vi "get leafnodes for traverse.vi"(8 "error in":errorcluster caption="错误输入（无错误）", 10 "Data in":refnum<data-value>[](array[refnum]), 11 "Class in":refnum<class "PanelLinkNode.lvclass"> caption="DNL_LabVIEW Object in") -> (0 "error out":errorcluster caption="错误输出", 2 "Data out":refnum<data-value>[](array[refnum]), 3 "Class out":refnum<class "PanelLinkNode.lvclass"> caption="DNL_LabVIEW Object out")   [LabVIEW 2013, in "PanelLinkNode.lvclass"]
uses:
  PanelLinkNode.lvclass
  PanelObject/PanelObject.lvclass
  PanelLinkNode.lvclass/PanelLinkNode.ctl
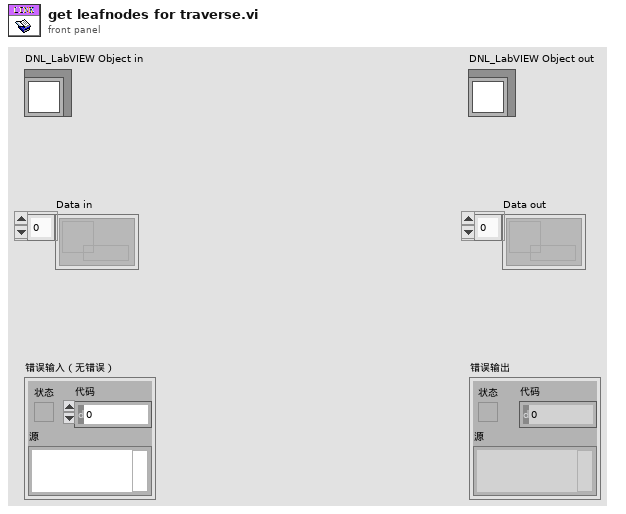
[diagram p1: front panel]
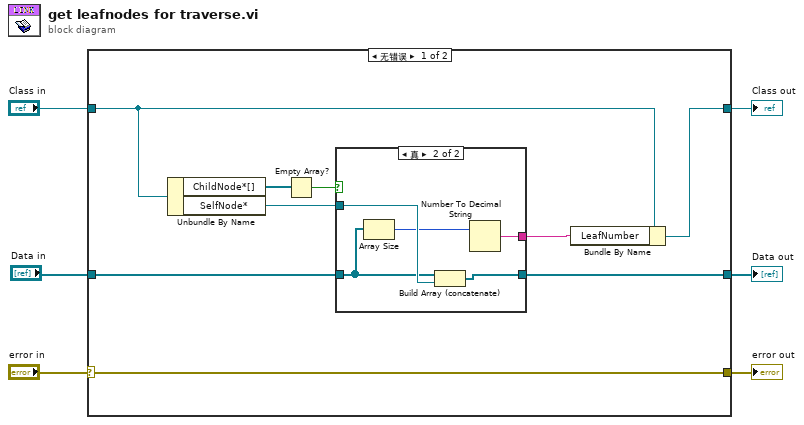
[diagram p0: block diagram]
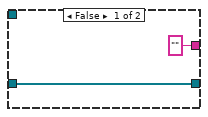
[diagram p2: hidden frame]
diagram:
  n1 = case shown="无错误" "error in" {
    selector: "error in" -> [w15 w25]
    tunnel: [w15 w25] -> w5
    tunnel: [w7 w24] -> w3
    tunnel: "Class in" -> [w9 w24]
    tunnel: "Data in" -> [w12 w23]
    tunnel: [w10 w23] -> w1
    frame No Error {
      n2 = Unbundle By Name(w9) -> ("ChildNode*[]"=w14:refnum<data-value>[], "SelfNode*"=w11:refnum<data-value>)
      n3 = Empty Array?(array=w14) -> (empty?=w13:bool)
      n4 = case shown="真" w13 {
        tunnel: w12 -> [w17 w20]
        tunnel: w11 -> [_ w22]
        tunnel: [w17 w21] -> w10
        tunnel: ["" w18] -> w8
        frame False {
        }
        frame True {
          n5 = Array Size(array=w20) -> (size(s)=w19:i32)
          n6 = Build Array (concatenate)(w20, w22) -> (w21:refnum<data-value>[])
          n7 = Number To Decimal String(number=w19) -> (decimal integer string=w18:string)  [unwired: 1 in]
        }
      }
      n8 = Bundle By Name(cluster=w9, "LeafNumber"=w8) -> (w7:refnum<class "PanelLinkNode.lvclass">)
    }
    frame Error {
    }
  }
  "error out" <- w5
  "Class out" <- w3
  "Data out" <- w1
